vi "Read ini file.vi"(0 "input string":string, 1 "SEQ":i32) -> (3 "Array":string[](array[string]), 5 "Item":string)   [LabVIEW 2018]
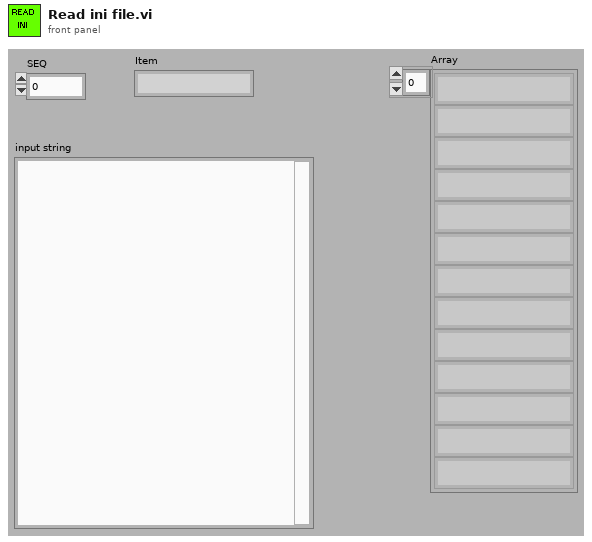
[diagram p1: front panel]
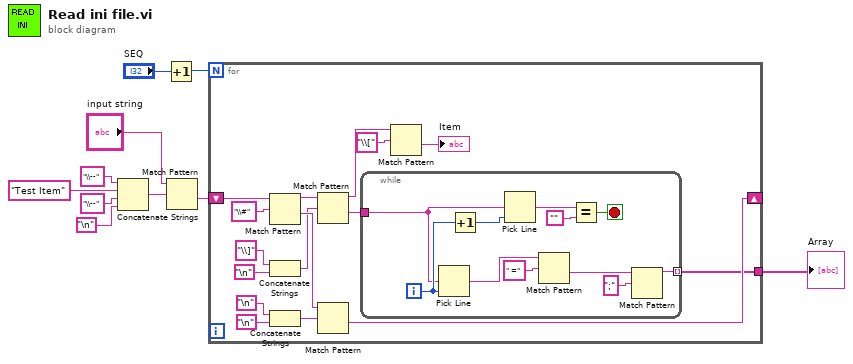
[diagram p0: block diagram]
diagram:
  n1 = Concatenate Strings("\\--" ("regular expression"), "Test Item" ("string"), "\\--" ("string"), "\n") -> (w10:string)
  n2 = Increment(x="SEQ") -> (x+1=w4:i32)
  n3 = Match Pattern(string="input string", regular expression=w10) -> (after substring=w5:string)  [unwired: 4 out]
  n4 = for {
    N: w4 -> [_]
    shift-right: [w20] -> _
    shift-left: w5 -> [w25]
    tunnel: [w11] -> w1
    n5 = Match Pattern(string=w25, regular expression="\\#") -> (before substring=w19:string, after substring=w21:string)  [unwired: 3 out]
    n6 = Concatenate Strings("\\]" ("regular expression"), "\n") -> (w15:string)
    n7 = Concatenate Strings("\n", "\n") -> (w22:string)
    n8 = Match Pattern(string=w19, regular expression=w15) -> (before substring=w14:string, after substring=w18:string)  [unwired: 3 out]
    n9 = Match Pattern(string=w21, regular expression=w22) -> (after substring=w20:string)  [unwired: 4 out]
    n10 = while {
      tunnel: w18 -> [w27]
      tunnel: [w28] -> w11 mode=indexing
      i -> [w34]
      stop <- w36 stop-if-true
      n11 = Pick Line(multi-line string=w27, line index=w34) -> (output string=w29:string)  [unwired: 1 out]
      n12 = Increment(x=w34) -> (x+1=w35:i32)
      n13 = Pick Line(multi-line string=w27, line index=w35) -> (output string=w33:string)  [unwired: 1 out]
      n14 = Match Pattern(string=w29, regular expression=" =") -> (after substring=w31:string)  [unwired: 4 out]
      n15 = Equal?(x=w33, y="") -> (x = y?=w36:bool)
      n16 = Match Pattern(string=w31, regular expression=";") -> (before substring=w28:string)  [unwired: 4 out]
    }
    n17 = Match Pattern(string=w14, regular expression="\\[") -> (after substring=→"Item":string)  [unwired: 4 out]
  }
  "Array" <- w1
